vi "EstimateVelocity&Angle.vi"(9 "Circle variables in":T3={"v_estimated_0"=[0.0, 0.0, 0.0, 0.0, 0.0], "Pose0 (X, Y, Theta)"=[0.0, 0.0, 0.0], "Omega_0"=[0.0, 0.0, 0.0, 0.0, 0.0], "time0"=0.0}, 10 "time":dbl, 11 "Pose (X, Y, Theta)":dbl[](array[numeric])=[0.0, 0.0, 0.0]) -> (3 "Estimated values":T2, 8 "Circle variables out":T1={"v_estimated"=[0.00033152226159632907+0.0i, 0.0+0.0i, 0.0+0.0i, 0.0+0.0i, 0.0+0.0i], "Pose (X, Y, Theta) out"=[-1.61394543457, 1.02296868896, -121.953392029], "OmegaUt"=[-0.021158443978342874, 0.0, 0.0, 0.0, 0.0], "time"=5763.816666})   [LabVIEW 2013]
uses:
  <vilib>/imath/engines/lvmath2/RunTimeEngine/ErrorHandling/NIMS_Finalize Error.vi
  <vilib>/imath/engines/lvmath2/RunTimeEngine/Managers/WorkSpace/UID Generator.vi
  <vilib>/imath/engines/lvmath2/RunTimeEngine/Managers/SymbolTable/Clear UID.vi
  <vilib>/imath/engines/lvmath2/RunTimeEngine/NodeEndStatement/NIMS_NodeEndStatement_Output.vi
  <instcachedir>/0/NIMS_NodeEndStatement_Output_53EC0D466D134D7ABD903AC30B43404B.lvgen/NIMS_NodeEndStatement_Output_53EC0D466D134D7ABD903AC30B43404B_010.vi
  <instcachedir>/0/NIMS_NodeEndStatement_Output_53EC0D466D134D7ABD903AC30B43404B.lvgen/NIMS_NodeEndStatement_Output_53EC0D466D134D7ABD903AC30B43404B_001.vi
  <instcachedir>/0/NIMS_NodeEndStatement_Output_53EC0D466D134D7ABD903AC30B43404B.lvgen/NIMS_NodeEndStatement_Output_53EC0D466D134D7ABD903AC30B43404B_009.vi
  <instcachedir>/0/NIMS_NodeEndStatement_Output_53EC0D466D134D7ABD903AC30B43404B.lvgen/NIMS_NodeEndStatement_Output_53EC0D466D134D7ABD903AC30B43404B_005.vi
  <instcachedir>/0/NIMS_NodeEndStatement_Output_53EC0D466D134D7ABD903AC30B43404B.lvgen/NIMS_NodeEndStatement_Output_53EC0D466D134D7ABD903AC30B43404B_000.vi
  <vilib>/imath/engines/lvmath2/RunTimeEngine/RunTimeType/NIMS_RunTimeType_From StrictType (excl LVString).vi
  <instcachedir>/0/NIMS_RunTimeType_From StrictType (excl LVString)_4DEE718D6EB74582AA20236969C084FC.lvgen/NIMS_RunTimeType_From StrictType (excl LVString)_4DEE718D6EB74582AA20236969C084FC_000.vi
  <vilib>/imath/engines/lvmath2/RunTimeEngine/LocalVariableDefStatement/MC_LocalVariableDefStatement_Display.vi
  <vilib>/imath/engines/lvmath2/RunTimeEngine/IndexRead/NIMS V(S).vi
  <instcachedir>/0/NIMS V(S)_0488751826AF41519A22953C041130DC.lvgen/NIMS V(S)_0488751826AF41519A22953C041130DC_000.vi
  <vilib>/imath/engines/lvmath2/RunTimeEngine/BuiltInFunctions/is_nan/NIMS_is_nan.vi
  <instcachedir>/0/NIMS_is_nan_BCCD798162CC49E3A8E57072444F6EB6.lvgen/NIMS_is_nan_BCCD798162CC49E3A8E57072444F6EB6_002.vi
  <vilib>/imathl/engines/lvmath/Functions/Error Handling/Create Error.vi
  <vilib>/imath/engines/lvmath2/RunTimeEngine/ErrorHandling/NIMS_Create Error From Enums.vi
  <vilib>/imath/engines/lvmath2/RunTimeEngine/BuiltInFunctions/length/NIMS_length(GV).vi
  <instcachedir>/0/NIMS_length(GV)_08A3D13377FD4E4B96F5795FBF3698FA.lvgen/NIMS_length(GV)_08A3D13377FD4E4B96F5795FBF3698FA_000.vi
  <vilib>/imath/engines/lvmath2/RunTimeEngine/IndexRead/NIMS V(R2).vi
  <instcachedir>/0/NIMS V(R2)_C76619605A0E4E9F8B2FA9389712AC47.lvgen/NIMS V(R2)_C76619605A0E4E9F8B2FA9389712AC47_000.vi
  <vilib>/imath/engines/lvmath2/RunTimeEngine/BuiltInFunctions/median/NIMS_CS=median(CV,I32).vi
  <vilib>/imath/engines/lvmath2/RunTimeEngine/ErrorHandling/NIMS_Error From Error Code.vi
  <vilib>/imath/engines/lvmath2/RunTimeEngine/BuiltInFunctions/median/NIMS_RS=median(RV,I32).vi
  <vilib>/imath/engines/lvmath2/RunTimeEngine/BuiltInFunctions/atan/NIMS_atan(C).vi
  <instcachedir>/0/NIMS_atan(C)_7C2C2596D2F04E9E823B85B74D765718.lvgen/NIMS_atan(C)_7C2C2596D2F04E9E823B85B74D765718_001.vi
  <vilib>/imath/engines/lvmath2/RunTimeEngine/Managers/SymbolTable/NIMS_WorkSpace.lvlib
panel:
  out "hejsan":i32
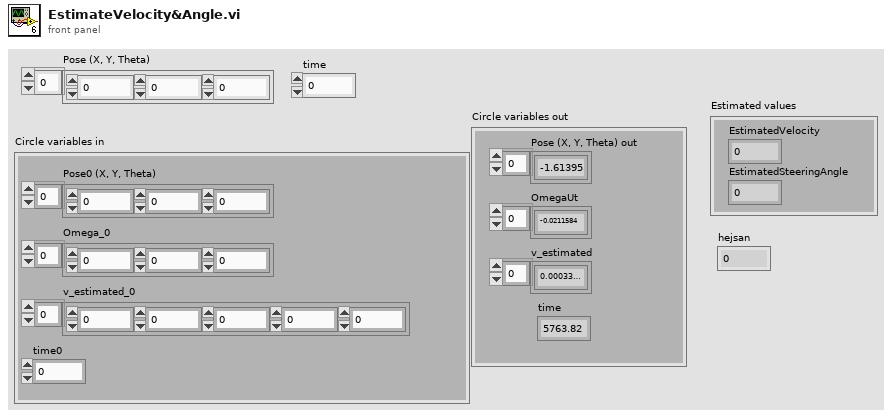
[diagram p1: front panel]
types:
  T1 = cluster{"v_estimated":cdb[], "Pose (X, Y, Theta) out":dbl[], "OmegaUt":dbl[], "time":dbl}
  T2 = cluster{"EstimatedVelocity":cdb, "EstimatedSteeringAngle":cdb}
  T3 = cluster{"v_estimated_0":dbl[], "Pose0 (X, Y, Theta)":dbl[], "Omega_0":dbl[], "time0":dbl}
  T4 = cluster{"v_estimated":cdb[], "Pose (X, Y, Theta)":dbl[], "OmegaUt":dbl[], "time":dbl}
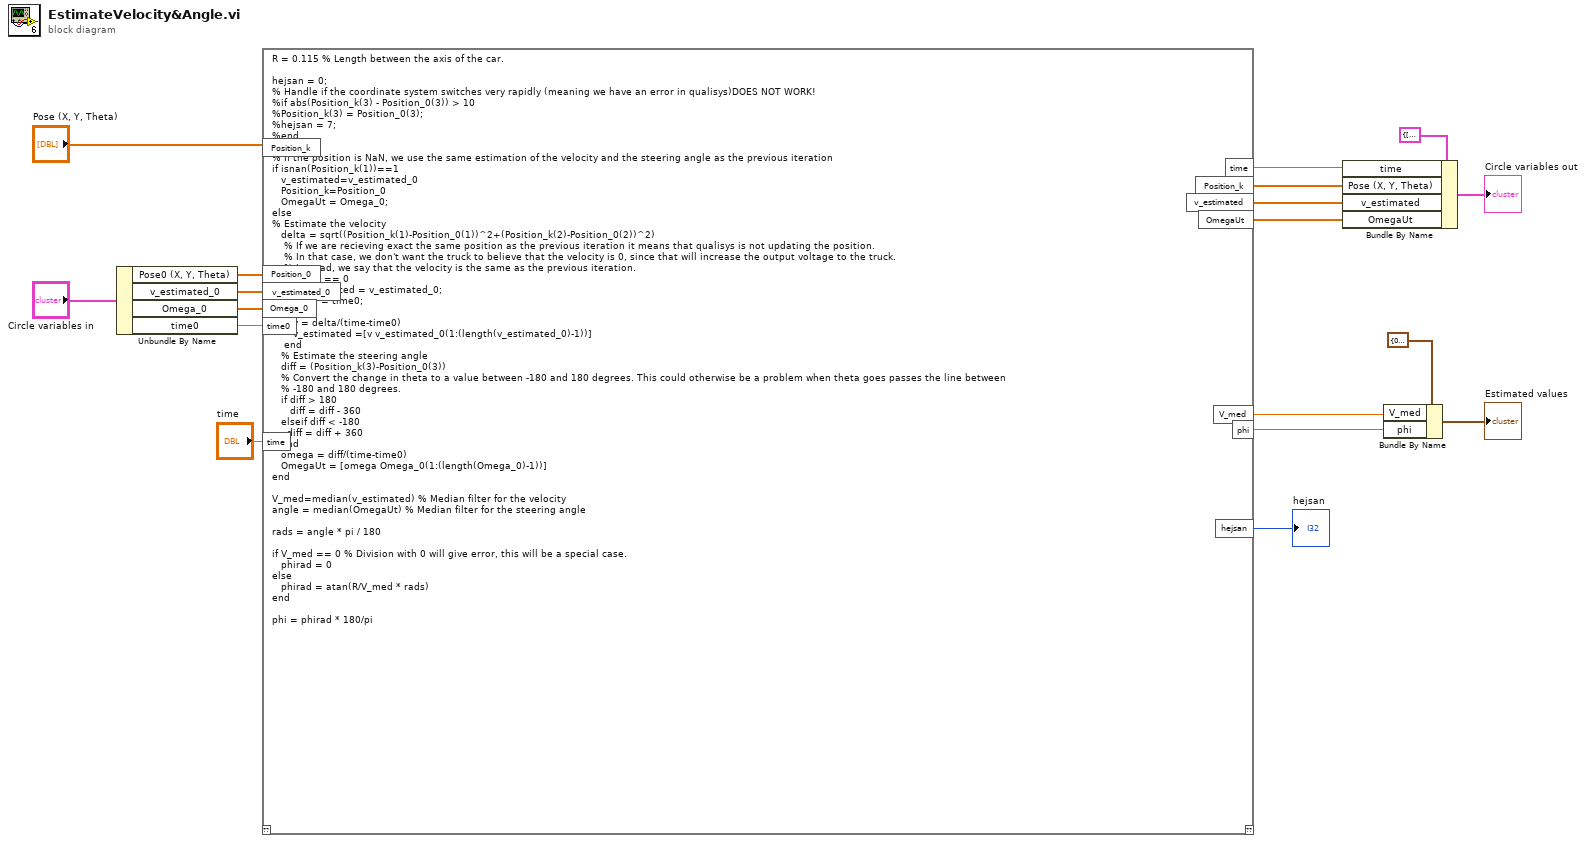
[diagram p0: block diagram]
diagram:
  n1 = Unbundle By Name("Circle variables in") -> ("Pose0 (X, Y, Theta)"=w12:dbl[], "v_estimated_0"=w11:dbl[], "Omega_0"=w10:dbl[], "time0"=w9:dbl)
  n2 = mathscript code="R = 0.115 % Length between the axis of the car.\n\nhejsan = 0;\n% Handle if the coordinate system switches very rapidly (meaning we have an error in qualisys)DOES NOT WORK!\n%if abs(Position_k(3) - Position_0(3)) > 10\n%Position_k(3) = Position_0(3);\n%hejsan = 7;\n%end\n\n% If the position is NaN, we use the same estimation of the velocity and the steering angle as the previous iteration\nif isnan(Position_k(1))==1\n   v_estimated=v_estimated_0\n   Position_k=Position_0\n   OmegaUt = Omega_0;\nelse\n% Estimate the velocity\n   delta = sqrt((Position_k(1)-Position_0(1))^2+(Position_k(2)-Position_0(2))^2)\n    % If we are recieving exact the same position as the previous iteration it means that qualisys is not updating the position.\n    % In that case, we don't want the truck to believe that the velocity is 0, since that will increase the output voltage to the truck.\n    % Instead, we say that the velocity is the same as the previous iteration.\n     if delta == 0\n        v_estimated = v_estimated_0;\n        time = time0;\n    else\n       v = delta/(time-time0)\n       v_estimated =[v v_estimated_0(1:(length(v_estimated_0)-1))]\n    end\n   % Estimate the steering angle\n   diff = (Position_k(3)-Position_0(3))\n   % Convert the change in theta to a value between -180 and 180 degrees. This could otherwise be a problem when theta goes passes the line between\n   % -180 and 180 degrees.\n   if diff > 180\n      diff = diff - 360\n   elseif diff < -180\n     diff = diff + 360\n   end\n   omega = diff/(time-time0)\n   OmegaUt = [omega Omega_0(1:(length(Omega_0)-1))]\nend\n\nV_med=median(v_estimated) % Median filter for the velocity\nangle = median(OmegaUt) % Median filter for the steering angle\n\nrads = angle * pi / 180\n\nif V_med == 0 % Division with 0 will give error, this will be a special case.\n   phirad = 0\nelse\n   phirad = atan(R/V_med * rads)\nend\n \nphi = phirad * 180/pi"("Position_k"="Pose (X, Y, Theta)", "Position_0"=w12, "time0"=w9, "v_estimated_0"=w11, "Omega_0"=w10, "time"="time") -> ("Position_k"=w8:dbl[], "v_estimated"=w7:cdb[], "V_med"=w5:cdb, "OmegaUt"=w6:dbl[], "phi"=w4:cdb, "time"=w2:dbl, "hejsan"=→"hejsan":i32)  [unwired: 1 in, 1 out]
  n3 = Bundle By Name(cluster=T4 {"v_estimated"=[], "Pose (X, Y, Theta)"=[], "OmegaUt"=[], "time"=0.0} ("Circle variables out"), "time"=w2, "Pose (X, Y, Theta)"=w8, "v_estimated"=w7, "OmegaUt"=w6) -> (→"Circle variables out":T4)
  n4 = Bundle By Name(cluster=cluster{"V_med":cdb, "phi":cdb} {"V_med"=0.0+0.0i, "phi"=0.0+0.0i} ("Display"), "V_med"=w5, "phi"=w4) -> (→"Estimated values":cluster{"V_med":cdb, "phi":cdb})
